vi "gfitsio-read-key-double.vi"(7 "keyname":string, 8 "error in (no error)":errorcluster, 9 "default value":dbl, 11 "gfits refnum":T1) -> (0 "error out":errorcluster, 1 "comment":string, 2 "value":dbl, 3 "dup gfits refnum":T1, 4 "units":string)   [LabVIEW 2011, in "gfitsio.lvlib"]
doc: "Return the specified keyword. <B>default value</B> specifies the desired returned data type of the keyword value. Data type conversion will be performed for numeric values if the keyword value does not have the same data type. If the keyword does not exist or an error occurs <B>value</B> will be equal to <B>default value</B>."
uses:
  gfitsio.lvlib
  gfitsio-refnum.ctl
  cfitsio-hdutypes.ctl
  gfitsio.dll
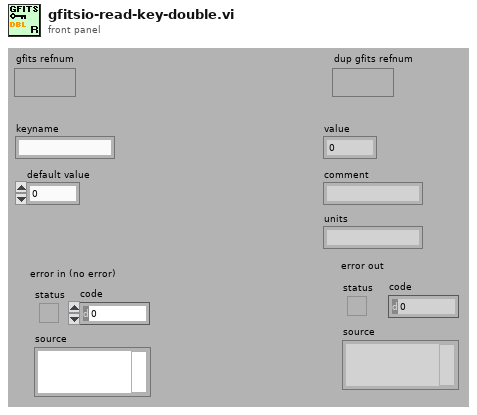
[diagram p1: front panel]
types:
  T1 = typedef "gfitsio.lvlib/gfitsio-refnum.ctl" = refnum<k1>
  T2 = typedef "gfitsio.lvlib/cfitsio-hdutypes.ctl" = i32
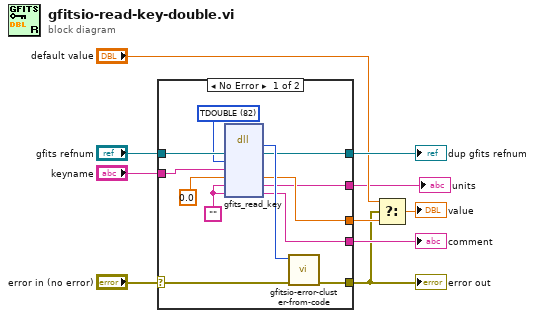
[diagram p0: block diagram]
diagram:
  n1 = case shown="No Error" "error in (no error)" {
    selector: "error in (no error)" -> [w21 w24]
    tunnel: [w20 w24] -> w4
    tunnel: "gfits refnum" -> [w18 w23]
    tunnel: [w19 w23] -> w9
    tunnel: "keyname" -> [w16 _]
    tunnel: [w14 _] -> w5
    tunnel: [w12 _] -> w6
    tunnel: [w13 _] -> w1
    frame No Error {
      w11 = ""
      w17 = T2 82 items=["TBIT"=1, "TBYTE  (U8)"=11, "TSBYTE  (I8)"=12, "TLOGICAL"=14, "TSTRING"=16, "TUSHORT  (U16)"=20, "TSHORT  (I16)"=21, "TUINT"=31, "TULONG  (U32)"=40, "TLONG  (I32)"=41, "TFLOAT  (SGL)"=42, "TLONGLONG  (I64)"=81, "TDOUBLE"=82, "TCOMPLEX  (CSG)"=83, "TDOUBLECOMPLEX  (CDB)"=163] ("cfitsio datatype")
      n2 = dll-call lib="C:/BonOMM/BonOMM-SAOMM/SubVIs/gfitsio/gfitsio.dll" fn="gfits_read_key"("gfits refnum"=w18, "datatype"=w17, "keyname"=w16, "value"=0.0, "units"=w11, "comment"=w11) -> (w22:i32, "gfits refnum"=w19:T1, "value"=w14:dbl, "units"=w13:string, "comment"=w12:string)  [unwired: 5 in, 2 out]
      n3 = call "gfitsio-error-cluster-from-code.vi"("error in (no error)"=w21, "error code"=w22) -> ("error out"=w20:errorcluster)  [unwired: 9 in]
    }
    frame Error {
    }
  }
  "error out" <- w4
  "dup gfits refnum" <- w9
  "comment" <- w6
  "units" <- w1
  n4 = Select(t="default value", s=w4, f=w5) -> (s? t:f=→"value":dbl)
